vi "svc_Get X-Axis Strings.vi"(1 "x-axis units":T1 items=["Time (s)"=0, "Frequency-CB (Hz)"=1, "Frequency-CPB (Hz)"=1248, "Frequency-Arbitrary (Hz)"=2357, "Quefrency (s)"=2, "Revolutions (rev)"=3, "Order"=4, "Speed (RPM)"=11, "Speed (rad/s)"=21, "Critical Band"=31, "Critical Band Rate (Bark)"=32, "None"=98, "Index"=65535]) -> (4 "x-axis label":string, 5 "x-axis unit string":string)   [LabVIEW 2017]
uses:
  <vilib>/addons/_NISVFA/_Shared subVIs/Controls/svc_X-Axis Units.ctl
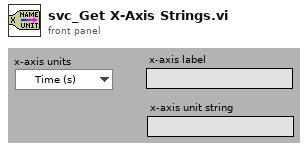
[diagram p1: front panel]
types:
  T1 = typedef "svc_X-Axis Units.ctl" = u16
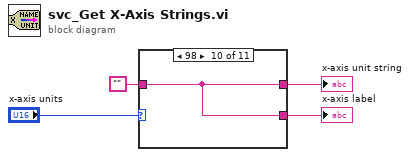
[diagram p0: block diagram]
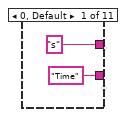
[diagram p2: hidden frame]
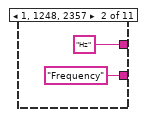
[diagram p3: hidden frame]
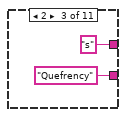
[diagram p4: hidden frame]
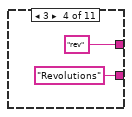
[diagram p5: hidden frame]
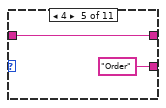
[diagram p6: hidden frame]
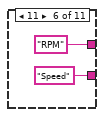
[diagram p7: hidden frame]
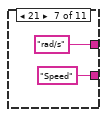
[diagram p8: hidden frame]
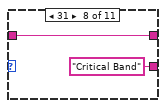
[diagram p9: hidden frame]
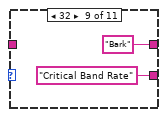
[diagram p10: hidden frame]
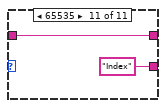
[diagram p11: hidden frame]
diagram:
  n1 = case shown="98" "x-axis units" {
    tunnel: ["Time" ("channel name") "Frequency" ("channel name") "Quefrency" ("channel name") "Revolutions" ("channel name") "Order" ("channel name") "Speed" ("channel name") "Speed" ("channel name") "Critical Band" ("channel name") "Critical Band Rate" w23 "Index" ("channel name")] -> w2
    tunnel: ["s" "Hz" "s" "rev" w13 "RPM" "rad/s" w20 "Bark" w23 w24] -> w1
    tunnel: "" -> [_ _ _ _ w13 _ _ w20 _ w23 w24]
    frame 0, Default {
    }
    frame 1, 1248, 2357 {
    }
    frame 2 {
    }
    frame 3 {
    }
    frame 4 {
    }
    frame 11 {
    }
    frame 21 {
    }
    frame 31 {
    }
    frame 32 {
    }
    frame 98 {
    }
    frame 65535 {
    }
  }
  "x-axis label" <- w2
  "x-axis unit string" <- w1
